vi "ReadQ.vi"(8 "error in (no error)":errorcluster) -> (0 "error out":errorcluster, 2 "Variant":variant, 3 "State":T1)   [LabVIEW 2017, in "Temp.lvlib"]
uses:
  Temp.lvlib
  ctl/MainStates.ctl
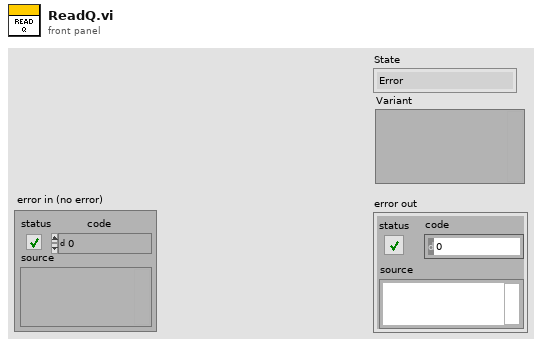
[diagram p1: front panel]
types:
  T1 = typedef "Temp.lvlib/MainStates.ctl" = enum16{"Error", "Exit", "Init"}
  T2 = typedef "Temp.lvlib/MainData.ctl" = cluster{"State":T1, "Variant":variant}
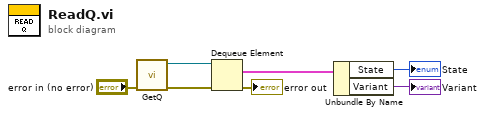
[diagram p0: block diagram]
diagram:
  n1 = call "GetQ.vi"("error in (no error)"="error in (no error)") -> ("error out"=w6:errorcluster, "Q out"=w7:refnum<queue>)  [unwired: 9 in]
  n2 = Dequeue Element(queue=w7, error in (no error)=w6) -> (element=w3:T2, error out=→"error out":errorcluster)  [unwired: 1 in, 2 out]
  n3 = Unbundle By Name(w3) -> ("State"=→"State":T1, "Variant"=→"Variant":variant)
